vi "JAG_Exercise2_Task1.vi"() -> ()   [LabVIEW 2014, in "Jacob_5th.lvrbt"]
uses:
  Jacob_5th/Jacob_5th.lvrbt
  <vilib>/NXT/Dual Mode Library/Display/drawText.vi
panel:
  out "Result":dbl
  out "A+B":dbl
  in  "B":dbl
  in  "A":dbl
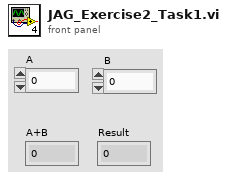
[diagram p1: front panel]
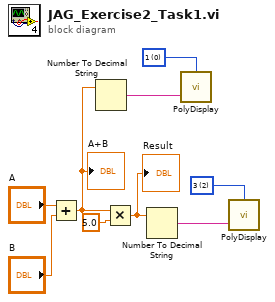
[diagram p0: block diagram]
diagram:
  w2 = i16 2 items=["1", "2", "3", "4", "5", "6", "7", "8", "9", "10", "11", "12"] ("Line")
  w4 = i16 0 items=["1", "2", "3", "4", "5", "6", "7", "8", "9", "10", "11", "12"] ("Line")
  n1 = Add(x="A", y="B") -> (x+y=w6:dbl)
  "A+B" <- w6
  n2 = Number To Decimal String(number=w6) -> (decimal integer string=w5:string)  [unwired: 1 in]
  n3 = Multiply(x=w6, y=5.0) -> (x*y=w1:dbl)
  "Result" <- w1
  n4 = Number To Decimal String(number=w1) -> (decimal integer string=w3:string)  [unwired: 1 in]
  n5 = call-poly <vilib>:"PolyDisplay.vi"("Text"=w5, "Line"=w4) -> ()  [unwired: 2 in, 1 out]
  n6 = call-poly <vilib>:"PolyDisplay.vi"("Text"=w3, "Line"=w2) -> ()  [unwired: 2 in, 1 out]
